vi "FFT_Complex.vi"(3 "Fs":dbl=2.0 format="%#_13g", 4 "Q":dbl[](array[numeric]), 5 "I":dbl[](array[numeric])) -> (0 "FFT Mag":dbl[](array[numeric]), 2 "FFT Freqs":dbl[](array[numeric]))   [LabVIEW 2024]
uses:
  <vilib>/Analysis/2dsp.llb/Complex FFT.vi
  <vilib>/Analysis/1siggen.llb/Ramp Pattern by Samples.vi
  <vilib>/Analysis/NI_AALPro.lvlib
  <vilib>/Analysis/NI_AALBase.lvlib
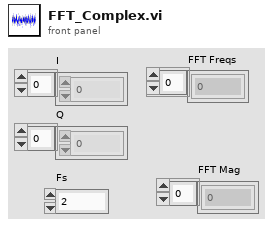
[diagram p1: front panel]
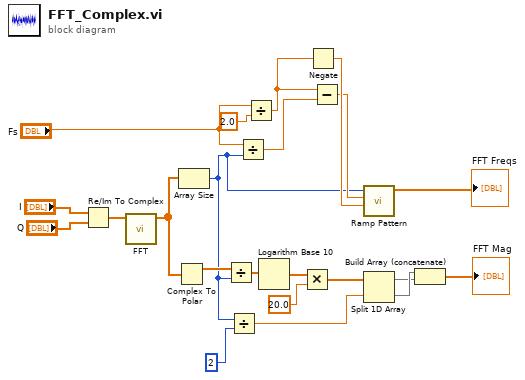
[diagram p0: block diagram]
diagram:
  n1 = Re/Im To Complex(1:"Q", 2:"I") -> (0:w20:cdb[])
  n2 = call-poly <vilib>:"FFT.vi"("X"=w20) -> ("FFT {X}"=w19:cdb[])  [unwired: 9 in, 1 out]
  n3 = Complex To Polar(r * e^(i*theta)=w19) -> (r=w15:dbl[])  [unwired: 1 out]
  n4 = Array Size(array=w19) -> (size(s)=w3:i32)
  n5 = Divide(x=w15, y=w3) -> (x/y=w14:dbl[])
  n6 = Divide(x=w3, y=2) -> (x/y=w1:dbl)
  n7 = Divide(x="Fs", y=w3) -> (x/y=w12:dbl)
  n8 = Divide(x="Fs", y=2.0) -> (x/y=w13:dbl)
  n9 = Logarithm Base 10(1:w14) -> (0:w17:dbl[])
  n10 = Multiply(x=w17, y=20.0) -> (x*y=w9:dbl[])
  n11 = Negate(x=w13) -> (-x=w11:dbl)
  n12 = Subtract(x=w13, y=w12) -> (x-y=w10:dbl)
  n13 = call-poly <vilib>:"Ramp Pattern.vi"("start"=w11, "end"=w10, "samples"=w3) -> ("Ramp Pattern"=→"FFT Freqs":dbl[])  [unwired: 7 in, 1 out]
  n14 = Split 1D Array(array=w9, index=w1) -> (first subarray=w7:dbl[], second subarray=w8:dbl[])
  n15 = Build Array (concatenate)(w8, w7) -> (→"FFT Mag":dbl[])
